vi "VI_folder_path.vi"() -> (0 "output path":path)   [LabVIEW 2015]
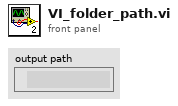
[diagram p1: front panel]
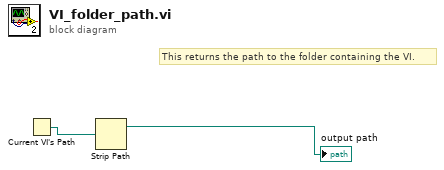
[diagram p0: block diagram]
diagram:
  # "This returns the path to the folder containing the VI."
  n1 = Current VI's Path() -> (path=w2:path)
  n2 = Strip Path(path=w2) -> (stripped path=→"output path":path)  [unwired: 1 out]
